vi "L01.vi"() -> ()   [LabVIEW 2020]
panel:
  in  "stop":bool
  out "Voltage Output":dbl
  in  "R2":dbl
  in  "R1":dbl
  in  "Voltage Input":dbl
  # "Adam Sokacz\n400177446\n3CC3 L01"
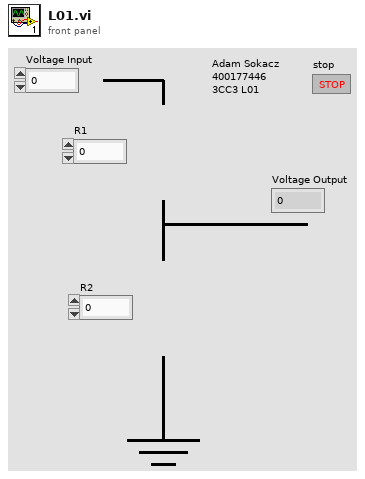
[diagram p1: front panel]
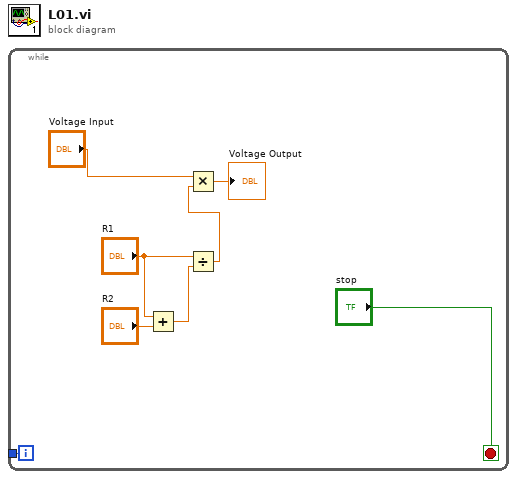
[diagram p0: block diagram]
diagram:
  n1 = while {
    tunnel: [w1] -> _
    i -> [w1]
    stop <- "stop" stop-if-true
    n2 = Add(x="R1", y="R2") -> (x+y=w6:dbl)
    n3 = Divide(x="R1", y=w6) -> (x/y=w5:dbl)
    n4 = Multiply(x="Voltage Input", y=w5) -> (x*y=→"Voltage Output":dbl)
  }
